vi "Write applicationElements.vi"(10 "applicationElements":T1, 11 "Model in":refnum<class "Model.lvclass">) -> (3 "Model out":refnum<class "Model.lvclass">)   [LabVIEW 2013, in "Model.lvclass"]
uses:
  Model.lvclass
  ApplicationElements/ApplicationElements.ctl
  ApplicationElements/DistanceGauge/DistanceGauge.lvclass
  ApplicationElements/ForceSensor/ForceSensor.lvclass
  ApplicationElements/SystemController/SystemController.lvclass
  ApplicationElements/StepperMotor/StepperMotor.lvclass
  ApplicationElements/TestMonitor/TestMonitor.lvclass
  ApplicationElements/Logger/Logger.lvclass
  ApplicationElements/Encoder/Encoder.lvclass
  ApplicationElements/StiffnessMonitor/StiffnessMonitor.lvclass
  ApplicationElements/Thermocouple/Thermocouple.lvclass
  Model.lvclass/Model.ctl
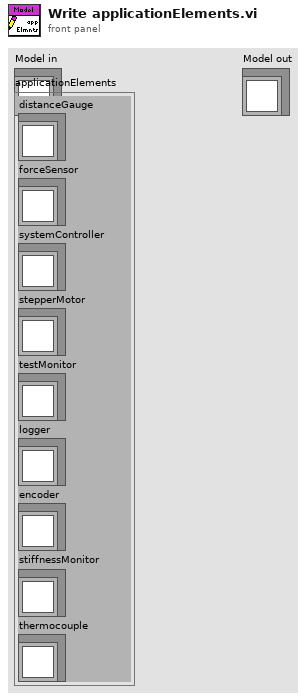
[diagram p1: front panel]
types:
  T1 = typedef "ApplicationElements.ctl" = cluster{"distanceGauge":refnum<class "DistanceGauge.lvclass">, "forceSensor":refnum<class "ForceSensor.lvclass">, "systemController":refnum<class "SystemController.lvclass">, "stepperMotor":refnum<class "StepperMotor.lvclass">, "testMonitor":refnum<class "TestMonitor.lvclass">, "logger":refnum<class "Logger.lvclass">, "encoder":refnum<class "Encoder.lvclass">, "stiffnessMonitor":refnum<class "StiffnessMonitor.lvclass">, "thermocouple":refnum<class "Thermocouple.lvclass">}
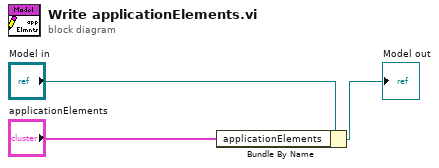
[diagram p0: block diagram]
diagram:
  n1 = Bundle By Name(cluster="Model in", "applicationElements"="applicationElements") -> (→"Model out":refnum<class "Model.lvclass">)
